vi "Keithley 4-wire probe.vi"(8 "error in (no error)":errorcluster, 11 "VISA resource name":refnum<visa-resource-name>) -> (0 "error out":errorcluster)   [LabVIEW 2018]
uses:
  <vilib>/Utility/file.llb/Write Delimited Spreadsheet (string).vi
  <vilib>/Utility/file.llb/Write Delimited Spreadsheet (DBL).vi
  Keithley 24XX.lvlib
panel:
  in  "write buffer":string="*RST\nFUNC \"RES\"\nRES:MODE AUTO\nRES:RANG 20E3\n:SYST:RSEN ON\n:FORM:ELEM RES\n:OUTP ON"
  out "Waveform Chart":dbl(graph)
  out "Resistance (ohms)":dbl
  out "Data string array":string[](array[string])
  out "read buffer":string
  out "error out 2":errorcluster
  out "Data numeric array":dbl[][](array[numeric])
  out "Time started":string
  out "List of times":dbl[](array[numeric])
  in  "file path (dialog if empty)":path
  in  "append to file? (new file:F)":bool=TRUE
  in  "wait time (sec)":u32
  in  "stop":bool
  out "time (sec)":dbl format="%_19f"
  # "4-point probe"
  # "sanity check"
  # "Put a number\nfor the resistance range.\nStart high and work your way down because \nthe higher the resistance range, the lower the source current."
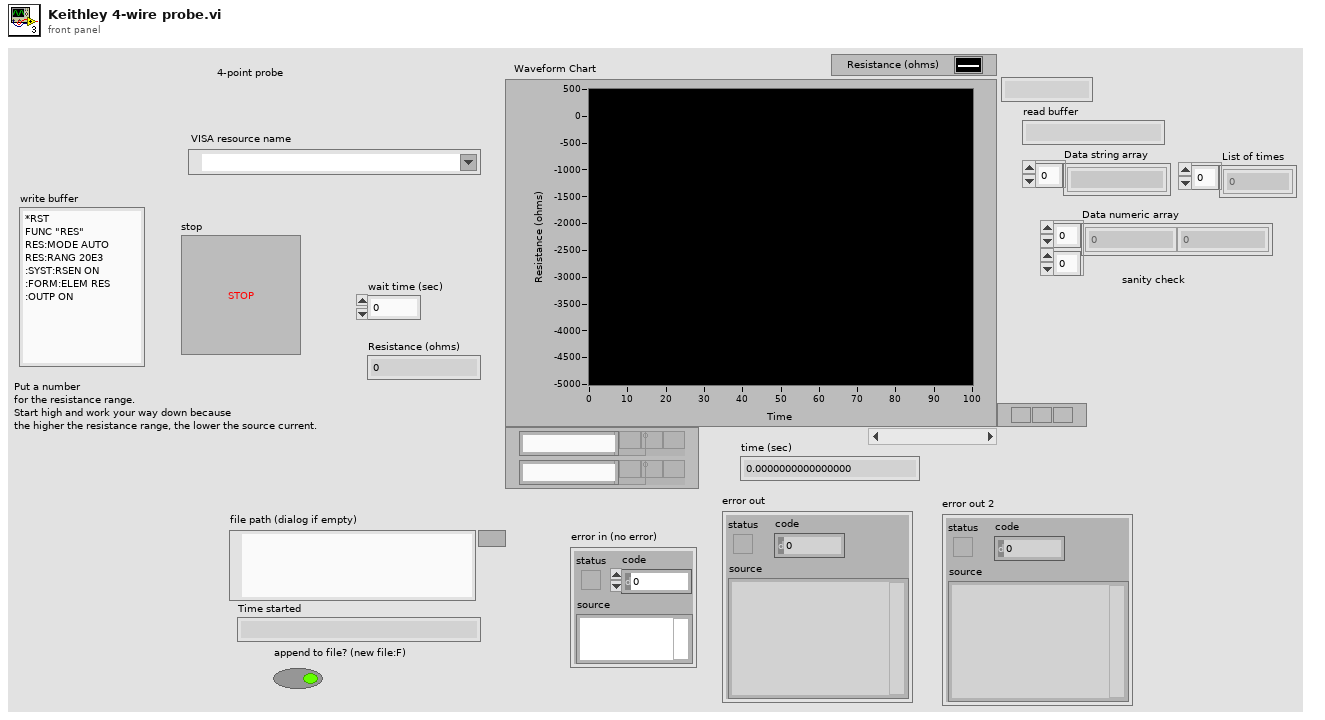
[diagram p1: front panel]
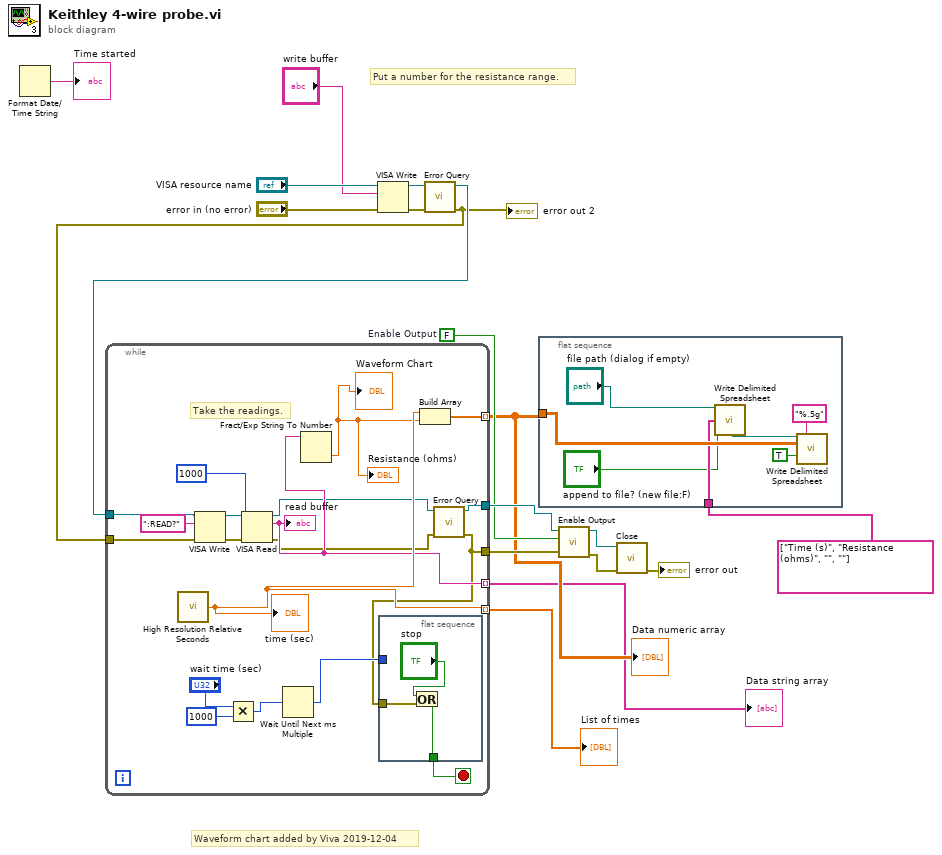
[diagram p0: block diagram]
diagram:
  w9 = FALSE  # Enable Output
  # "Put a number for the resistance range."
  # "Waveform chart added by Viva 2019-12-04"
  n1 = Format Date/Time String() -> (date/time string=→"Time started":string)  [unwired: 3 in]
  n2 = VISA Write(VISA resource name="VISA resource name", write buffer="write buffer", error in (no error)="error in (no error)") -> (VISA resource name out=w16:refnum<visa-resource-name>, error out=w15:errorcluster)  [unwired: 1 out]
  n3 = call "Error Query.vi"("error in (no error)"=w15, "VISA resource name"=w16) -> ("error out"=w2:errorcluster, "VISA resource name out"=w4:refnum<visa-resource-name>)  [unwired: 6 in, 2 out]
  "error out 2" <- w2
  n4 = while {
    tunnel: w2 -> [w29]
    tunnel: w4 -> [w30]
    tunnel: [w20] -> w13
    tunnel: [w21] -> w12
    tunnel: [w33] -> w8 mode=indexing
    tunnel: [w31] -> w7 mode=indexing
    tunnel: [w24] -> w1 mode=indexing
    stop <- w32 stop-if-true
    # "Take the readings."
    n5 = call <vilib>:"High Resolution Relative Seconds.vi"() -> ("relative seconds"=w31:dbl)
    "time (sec)" <- w31
    n6 = VISA Write(VISA resource name=w30, write buffer=":READ?", error in (no error)=w29) -> (VISA resource name out=w27:refnum<visa-resource-name>, error out=w26:errorcluster)  [unwired: 1 out]
    n7 = Multiply(x="wait time (sec)", y=u32 1000) -> (x*y=w35:u32)
    n8 = VISA Read(VISA resource name=w27, byte count=u32 1000, error in (no error)=w26) -> (VISA resource name out=w22:refnum<visa-resource-name>, read buffer=w24:string, error out=w23:errorcluster)  [unwired: 1 out]
    "read buffer" <- w24
    n9 = Wait Until Next ms Multiple(millisecond multiple=w35) -> (millisecond timer value=w34:u32)
    n10 = Fract/Exp String To Number(string=w24) -> (number=w19:dbl)  [unwired: 3 in, 1 out]
    "Resistance (ohms)" <- w19
    "Waveform Chart" <- w19
    n11 = flat-sequence {
      tunnel: w34 -> [_]
      tunnel: w20 -> [w39]
      tunnel: [w38] -> w32
      frame #0 {
        n12 = Or(x="stop", y=w39) -> (x .or. y?=w38:bool)
      }
    }
    n13 = Build Array(w31, w19) -> (w33:dbl[])
    n14 = call "Error Query.vi"("error in (no error)"=w23, "VISA resource name"=w22) -> ("error out"=w20:errorcluster, "VISA resource name out"=w21:refnum<visa-resource-name>)  [unwired: 6 in, 2 out]
  }
  "List of times" <- w7
  "Data numeric array" <- w8
  "Data string array" <- w1
  n15 = flat-sequence {
    tunnel: w8 -> [w47]
    tunnel: string[] ["Time (s)", "Resistance (ohms)", "", ""] ("Info header") -> [w42]
    frame #0 {
      n16 = call-poly <vilib>:"Write Delimited Spreadsheet.vi"("file path (dialog if empty)"="file path (dialog if empty)", "1D data"=w42, "append to file? (new file:F)"="append to file? (new file:F)") -> ("new file path (Not A Path if cancelled)"=w44:path)  [unwired: 11 in, 1 out]
      n17 = call-poly <vilib>:"Write Delimited Spreadsheet.vi"("file path (dialog if empty)"=w44, "format (%.3f)"="%.5g", "2D data"=w47, "append to file? (new file:F)"=TRUE) -> ()  [unwired: 10 in, 2 out]
    }
  }
  n18 = call "Enable Output.vi"("error in (no error)"=w13, "Enable Output (T: Enable)"=w9, "VISA resource name"=w12) -> ("error out"=w11:errorcluster, "VISA resource name out"=w10:refnum<visa-resource-name>)  [unwired: 7 in]
  n19 = call "Close.vi"("error in (no error)"=w11, "VISA resource name"=w10) -> ("error out"=→"error out":errorcluster)  [unwired: 9 in]
